vi "SIM ChkSimTimes.vi"(8 "Error In":errorcluster, 10 "finalTime":dbl, 11 "initialTime":dbl) -> (0 "Error Out":errorcluster)   [LabVIEW 2020]
uses:
  <vilib>/Simulation/Implementation/Shared/SIM Simulation Global Settings.vi
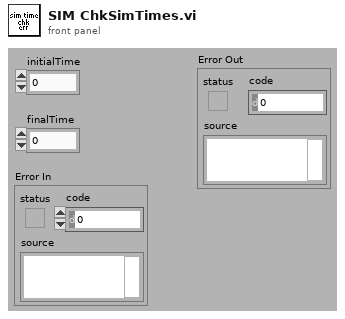
[diagram p1: front panel]
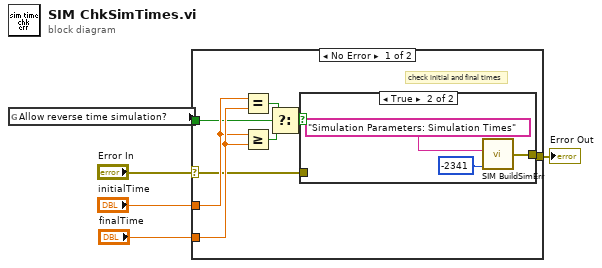
[diagram p0: block diagram]
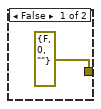
[diagram p2: hidden frame]
diagram:
  n1 = global read "SIM Simulation Global Settings.vi" "Allow reverse time simulation?"() -> (w3:bool)
  n2 = case shown="No Error" "Error In" {
    selector: "Error In" -> [w6 w18]
    tunnel: "finalTime" -> [w11 _]
    tunnel: "initialTime" -> [w10 _]
    tunnel: w3 -> [w8 _]
    tunnel: [w7 w18] -> w2
    frame No Error {
      # "check initial and final times"
      n3 = Equal?(x=w10, y=w11) -> (x = y?=w9:bool)
      n4 = Greater Or Equal?(x=w10, y=w11) -> (x >= y?=w12:bool)
      n5 = Select(t=w9, s=w8, f=w12) -> (s? t:f=w13:bool)
      n6 = case shown="True" w13 {
        tunnel: [errorcluster {"status"=FALSE, "code"=0, "source"=""} ("Error Cluster") w17] -> w7
        tunnel: w6 -> [_ _]
        frame False {
        }
        frame True {
          n7 = call <vilib>:"SIM BuildSimErr.vi"("error.code"=-2341, "Block Name"="Simulation Parameters: Simulation Times" ("CallChain")) -> ("Error Cluster"=w17:errorcluster)  [unwired: 2 in]
        }
      }
    }
    frame Error {
    }
  }
  "Error Out" <- w2
